vi "Write.vi"(8 "error in (no error)":errorcluster, 10 "Data":string, 11 "TcpClient in":refnum<class "TcpClient.lvclass">) -> (0 "error out":errorcluster, 3 "TcpClient out":refnum<class "TcpClient.lvclass">)   [LabVIEW 2022 SP3, in "TcpSocket.lvlib" / "TcpClient.lvclass"]
uses:
  TcpClient.lvclass
  TcpClient.lvclass/TcpClient.ctl
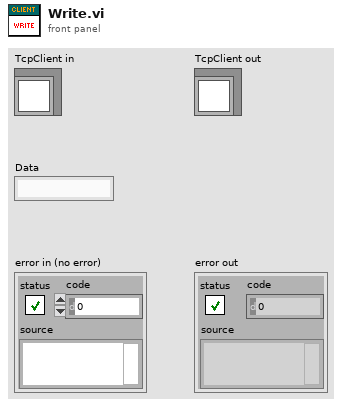
[diagram p1: front panel]
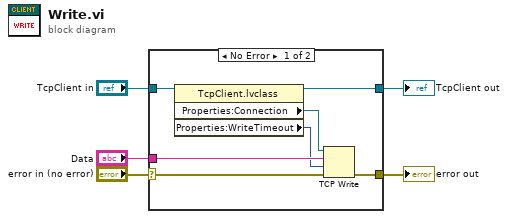
[diagram p0: block diagram]
diagram:
  n1 = case shown="No Error" "error in (no error)" {
    selector: "error in (no error)" -> [w12 w14]
    tunnel: [w11 w14] -> w4
    tunnel: [w8 w13] -> w2
    tunnel: "TcpClient in" -> [w10 w13]
    tunnel: "Data" -> [w9 _]
    frame No Error {
      n2 = property class="TcpClient.lvclass"(reference=w10) -> (reference out=w8:refnum<class "TcpClient.lvclass">, "Properties:Connection"=w6:refnum<k5>, "Properties:WriteTimeout"=w7:i32)  [unwired: 1 in, 1 out]
      n3 = TCP Write(connection ID=w6, data in=w9, error in (no error)=w12, 9:w7) -> (error out=w11:errorcluster)  [unwired: 2 out]
    }
    frame Error {
    }
  }
  "error out" <- w4
  "TcpClient out" <- w2
